vi "Destroy.vi"(8 "error in (no error)":errorcluster, 11 "User Interface Events in":refnum<class "User Interface Events.lvclass">) -> (0 "error out":errorcluster, 3 "User Interface Events out":refnum<class "User Interface Events.lvclass">)   [LabVIEW 2017, in "DSF Core.lvlib" / "User Interface Events.lvclass"]
uses:
  User Interface Events.lvclass
  User Interface Events.lvclass/User Interface Events.ctl
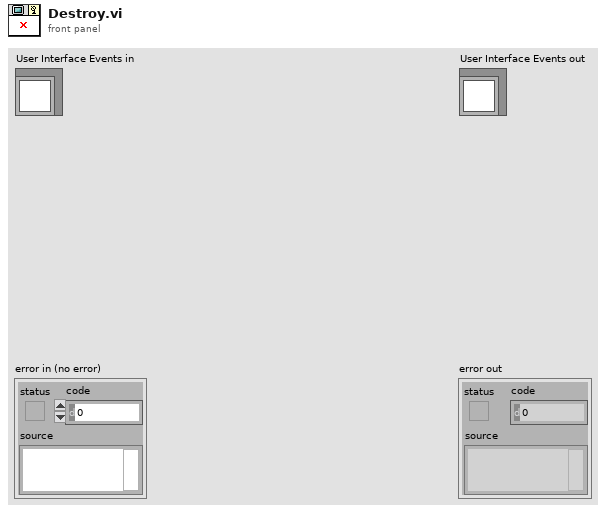
[diagram p1: front panel]
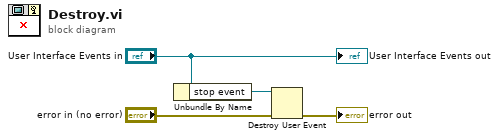
[diagram p0: block diagram]
diagram:
  n1 = Unbundle By Name("User Interface Events in") -> ("stop event"=w2:refnum<user-event>)
  n2 = Destroy User Event(user event=w2, error in="error in (no error)") -> (error out=→"error out":errorcluster)
  "User Interface Events out" <- "User Interface Events in"
